vi "VIMethodTemplate.vi"() -> (3 "VI out":refnum<vi>)   [LabVIEW 2021, in "YActor.lvclass"]
uses:
  YActor.lvclass
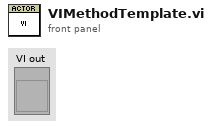
[diagram p1: front panel]
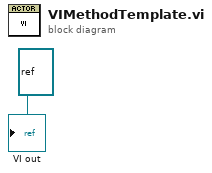
[diagram p0: block diagram]
diagram:
  "VI out" <- refnum<vi> refnum ("type specifier VI Refnum (for type only)")
